vi "Read Simulate Status.vi"(8 "error in (no error)":errorcluster, 11 "2575 in":refnum<class "2575.lvclass">) -> (0 "error out":errorcluster, 3 "2575 out":refnum<class "2575.lvclass">)   [LabVIEW 2019]
uses:
  2575.lvclass
  Desktop/Built/Configuration.lvlibp/Configuration.lvclass
  C:/Users/rdexter/Desktop/Built/SwitchMatrix.lvlibp/SwitchMatrix.lvclass
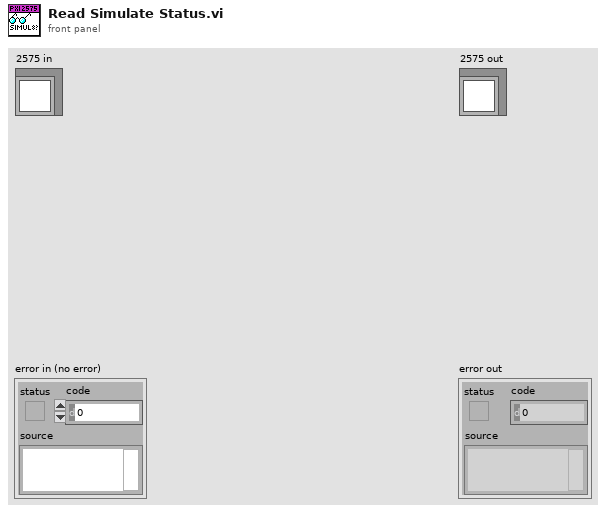
[diagram p1: front panel]
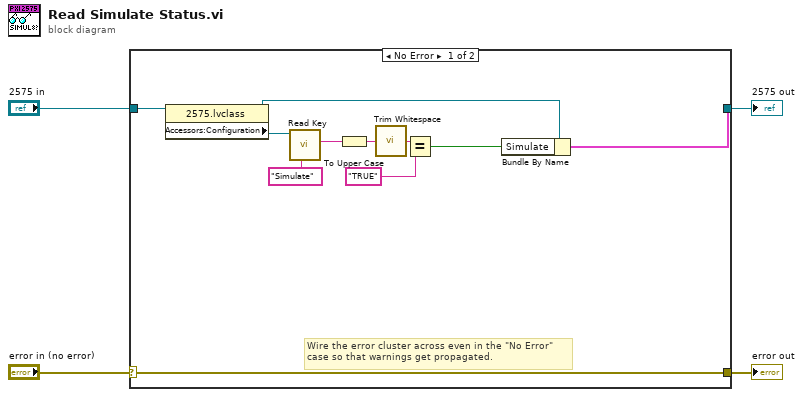
[diagram p0: block diagram]
diagram:
  n1 = case shown="No Error" "error in (no error)" {
    selector: "error in (no error)" -> [w14 w17]
    tunnel: [w14 w17] -> w3
    tunnel: [w6 w16] -> w1
    tunnel: "2575 in" -> [w15 w16]
    frame No Error {
      # "Wire the error cluster across even in the \"No Error\"\ncase so that warnings get propagated."
      n2 = property class="2575.lvclass"(reference=w15) -> (reference out=w13:refnum<class "2575.lvclass">, "Accessors:Configuration"=w12:refnum<class "Configuration.lvclass">)  [unwired: 1 in, 1 out]
      n3 = call "Read Key.vi"("Key Name"="Simulate", "Configuration in"=w12) -> ("Key Value"=w10:string)  [unwired: 7 in, 2 out]
      n4 = To Upper Case(1:w10) -> (0:w9:string)
      n5 = call <vilib>:"Trim Whitespace.vi"("string"=w9) -> ("trimmed string"=w8:string)  [unwired: 1 in]
      n6 = Equal?(x=w8, y="TRUE") -> (x = y?=w5:bool)
      n7 = Bundle By Name(cluster=w13, "Simulate"=w5) -> (w6:cluster{})
    }
    frame Error {
    }
  }
  "error out" <- w3
  "2575 out" <- w1
